vi "iWorx - Respiration Belt.vi"() -> ()   [LabVIEW 2012]
uses:
  <vilib>/measure/NI_MAPro.lvlib
  <vilib>/Analysis/NI_AALBase.lvlib
  <vilib>/Analysis/baseanly.llb/Mean (DBL).vi
  <vilib>/DAQmx/read.llb/DAQmx Read (Analog 1D Wfm NChan NSamp).vi
  <vilib>/DAQmx/configure/timing.llb/DAQmx Timing (Sample Clock).vi
  <vilib>/measure/macond.llb/IIR Filter for 1 Chan.vi
  <vilib>/DAQmx/create/channels.llb/DAQmx Create Channel (AI-Voltage-Basic).vi
panel:
  in  "Log Info Button":bool
  in  "Reset Scale":bool
  in  "Stop":bool
  out "Inst Breath Rate":dbl format="%5.1f BPM"
  in  "Set Up":bool
  in  "High Threshold":dbl=0.0005 format="%.5g"
  out "Avg Breath Rate":dbl format="%5.1f BPM"
  in  "Low Threshold":dbl=-0.0005 format="%.5f"
  out "error out":errorcluster
  in  "Auto-Threshold":bool
  in  "Channel":u16(ring) items=["Channel 1", "Channel 2"]
  in  "Pause Button":bool
  in  "Snapshot":bool
  out "Waveform Chart":waveform(dbl)(graph)
  in  "Clear Chart":bool
  in  "Open Log":bool
  in  "Rescale Y":bool
  out "Raw Signal":dbl(knob) scale=-0.1..0.1
  # "iWorx - Respiration Belt - Data Logger"
  # "Sensor Input"
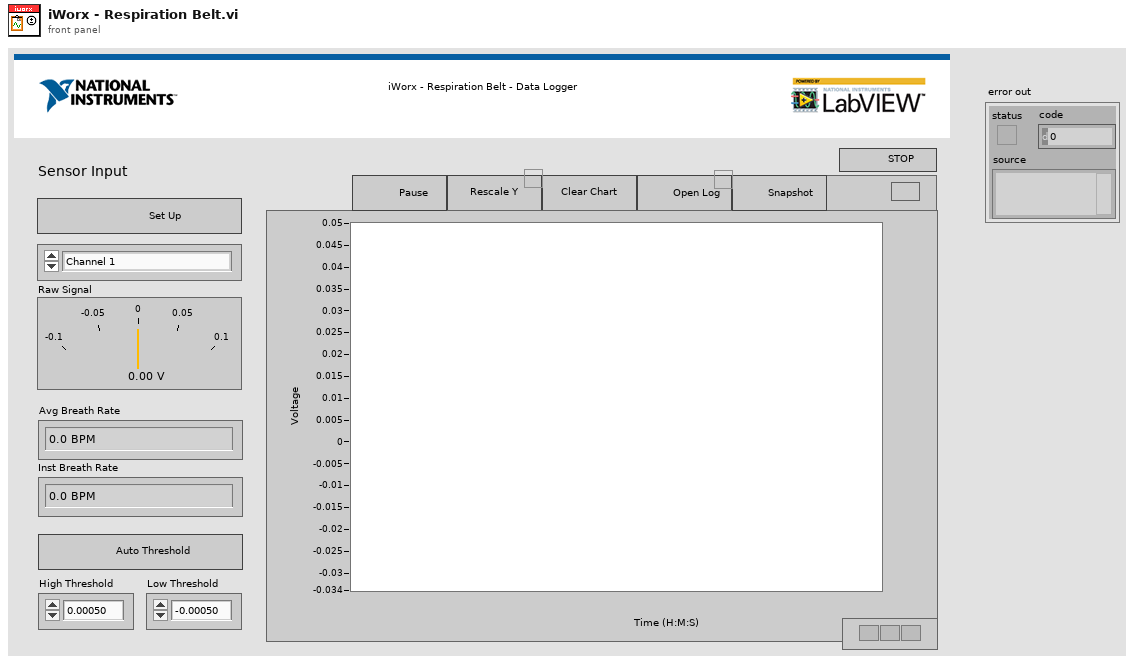
[diagram p1: front panel]
types:
  T1 = cluster{"Topology":enum16{"Off", "Butterworth", "Chebyshev", "Inverse Chebyshev", "Elliptic", "Bessel"}, "Type":enum16{"Lowpass", "Highpass", "Bandpass", "Bandstop"}, "Order":i32, "Lower Fc":dbl, "Upper Fc":dbl, "PB Ripple":dbl, "SB Attenuation":dbl}
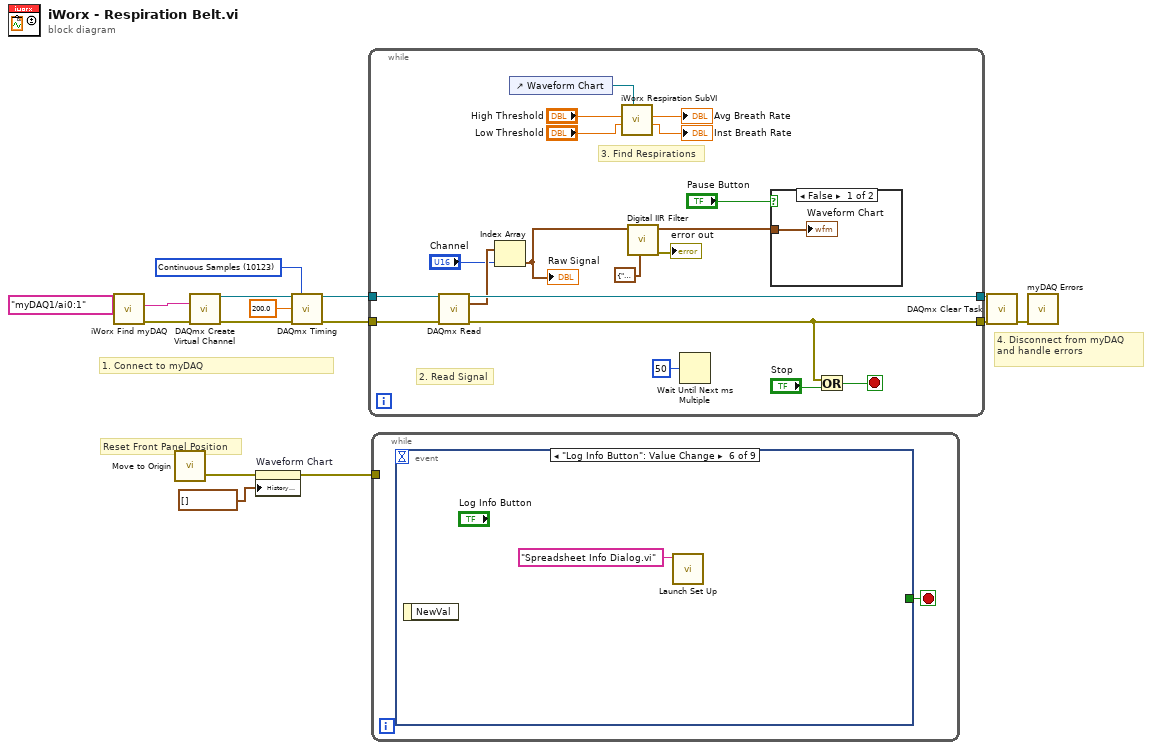
[diagram p0: block diagram]
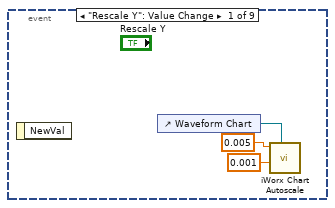
[diagram p2: hidden frame]
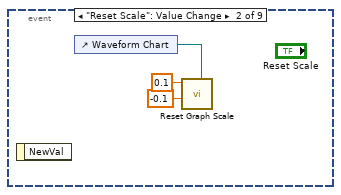
[diagram p3: hidden frame]
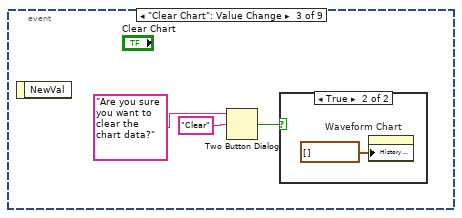
[diagram p4: hidden frame]
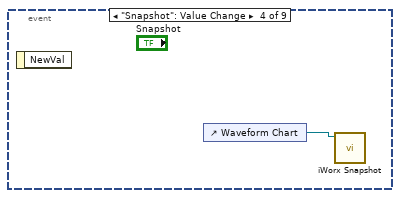
[diagram p6: hidden frame]
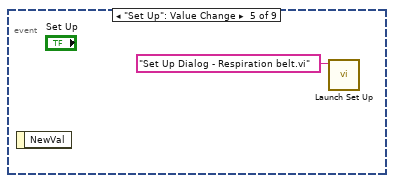
[diagram p7: hidden frame]
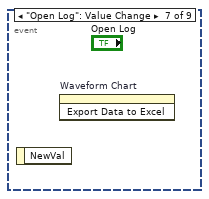
[diagram p8: hidden frame]
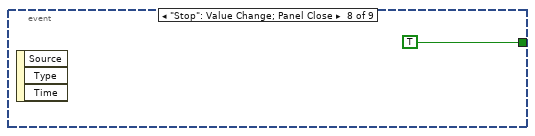
[diagram p9: hidden frame]
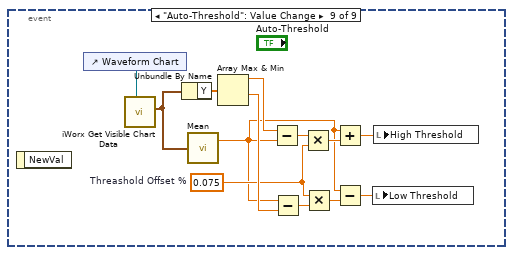
[diagram p10: hidden frame]
diagram:
  w7 = 10123 items=["Finite Samples"=10178, "Continuous Samples"=10123, "Hardware Timed Single Point"=12522] ("sample mode")
  # "Reset Front Panel Position"
  # "4. Disconnect from myDAQ and handle errors"
  # "1. Connect to myDAQ"
  n1 = call "iWorx Find myDAQ.vi"("Preferred myDAQ (myDAQ1)"=tag "myDAQ1/ai0:1" ("physical channels")) -> ("Error Out"=w3:errorcluster, "DAQmx Physical Channel"=w4:tag)  [unwired: 6 in, 3 out]
  n2 = call "Move to Origin.vi"() -> ("Error Out"=w2:errorcluster)  [unwired: 3 in]
  n3 = call-poly <vilib>:"DAQmx Create Virtual Channel.vi"("physical channels"=w4, "error in"=w3) -> ("task out"=w11:refnum<k21>, "error out"=w10:errorcluster)  [unwired: 12 in]
  n4 = property on="Waveform Chart" class="WFChart (strict)"(error in=w2, "History Data"=waveform(dbl)[] []) -> (error out=w13:errorcluster)  [unwired: 1 in, 1 out]
  n5 = call-poly <vilib>:"DAQmx Timing.vi"("task/channels in"=w11, "sample mode"=w7, "rate"=200.0, "error in"=w10) -> ("task out"=w8:refnum<k21>, "error out"=w9:errorcluster)  [unwired: 10 in]
  n6 = while {
    tunnel: w8 -> [w34]
    tunnel: [w33] -> w15
    tunnel: w9 -> [w32]
    tunnel: [w30] -> w14
    stop <- w31 stop-if-true
    # "3. Find Respirations"
    # "2. Read Signal"
    n7 = call-poly <vilib>:"DAQmx Read.vi"("task/channels in"=w34, "error in"=w32) -> ("task out"=w33:refnum<k21>, "data"=w28:waveform(dbl)[], "error out"=w30:errorcluster)  [unwired: 11 in]
    n8 = Index Array(array=w28, index="Channel") -> (element=w17:waveform(dbl))
    "Raw Signal" <- w17
    n9 = control-ref of="Waveform Chart"() -> (w22:refnum<vi>)
    n10 = call "iWorx Respiration SubVI.vi"("Waveform Chart"=w22, "low Threshold"="Low Threshold", "high Threshold"="High Threshold") -> ("Instantaneous Breath Rate"=→"Inst Breath Rate":dbl, "Avg Breaths per Minute"=→"Avg Breath Rate":dbl)  [unwired: 5 in, 2 out]
    n11 = call-poly <vilib>:"Digital IIR Filter.vi"("IIR filter specifications"=T1 {"Topology"=enum."Butterworth", "Type"=enum."Lowpass", "Order"=1, "Lower Fc"=1.0, "Upper Fc"=200.0, "PB Ripple"=1.0, "SB Attenuation"=60.0}, "signal in"=w17) -> ("error out"=→"error out":errorcluster, "signal out"=w23:waveform(dbl))  [unwired: 7 in, 1 out]
    n12 = Wait Until Next ms Multiple(millisecond multiple=u32 50) -> ()  [unwired: 1 out]
    n13 = case shown="False" "Pause Button" {
      tunnel: w23 -> [w35 _]
      frame False {
        "Waveform Chart" <- w35
      }
      frame True {
      }
    }
    n14 = Or(x=w30, y="Stop") -> (x .or. y?=w31:bool)
  }
  n15 = while {
    tunnel: w13 -> [_]
    stop <- w36 stop-if-true
    n16 = event shown="[5] \"Log Info Button\": Value Change" {
      selector: _ -> [_ _ _ _ _ _ _ _ _]
      dyn-events: _ -> [_ _ _ _ _ _ _ _ _]
      timeout: _ -> [_ _ _ _ _ _ _ _ _]
      tunnel: [_ _ _ _ _ _ _ TRUE _] -> w36
      event "Rescale Y": Value Change {
        n17 = event-data() -> ()  [unwired: 1 in, 1 out]
        n18 = control-ref of="Waveform Chart"() -> (w39:refnum<vi>)
        n19 = call "iWorx Chart Autoscale.vi"("Selection Chart"=w39, "Rounding Multiple (10)"=0.001 ("Rounding Multiple (1)"), "Min Range (1)"=0.005 ("Rounding Multiple (1)")) -> ()  [unwired: 6 in, 3 out]
      }
      event "Reset Scale": Value Change {
        n20 = event-data() -> ()  [unwired: 1 in, 1 out]
        n21 = control-ref of="Waveform Chart"() -> (w40:refnum<vi>)
        n22 = call "Reset Graph Scale.vi"("WaveformChart in"=w40, "Minimum (0)"=-0.1, "Maximum (100)"=0.1) -> ()  [unwired: 8 in, 1 out]
      }
      event "Clear Chart": Value Change {
        n23 = event-data() -> ()  [unwired: 1 in, 1 out]
        n24 = Two Button Dialog(message="Are you sure you want to clear the chart data?", 2:"Clear" ("T button name (\"OK\")")) -> (T button?=w44:bool)  [unwired: 1 in]
        n25 = case shown="True" w44 {
          frame False {
          }
          frame True {
            n26 = property on="Waveform Chart" class="WFChart (strict)"("History Data"=waveform(dbl)[] []) -> ()  [unwired: 2 in, 2 out]
          }
        }
      }
      event "Snapshot": Value Change {
        n27 = event-data() -> ()  [unwired: 1 in, 1 out]
        n28 = control-ref of="Waveform Chart"() -> (w47:refnum<vi>)
        n29 = call "iWorx Snapshot.vi"("WaveformChart in"=w47) -> ()  [unwired: 10 in, 1 out]
      }
      event "Set Up": Value Change {
        n30 = event-data() -> ()  [unwired: 1 in, 1 out]
        n31 = call "Launch Set Up.vi"("name or relative path"="Set Up Dialog - Respiration belt.vi") -> ()  [unwired: 9 in, 2 out]
      }
      event "Log Info Button": Value Change {
        n32 = event-data() -> ()  [unwired: 1 in, 1 out]
        n33 = call "Launch Set Up.vi"("name or relative path"="Spreadsheet Info Dialog.vi") -> ()  [unwired: 9 in, 2 out]
      }
      event "Open Log": Value Change {
        n34 = event-data() -> ()  [unwired: 1 in, 1 out]
        n35 = invoke on="Waveform Chart" class="WFChart (strict)" method="Export Data to Excel"() -> ()  [unwired: 3 in, 3 out]
      }
      event "Stop": Value Change; Panel Close {
        n36 = event-data() -> ()  [unwired: 1 in, 3 out]
      }
      event "Auto-Threshold": Value Change {
        w55 = 0.075  # Threashold Offset %
        n37 = event-data() -> ()  [unwired: 1 in, 1 out]
        n38 = control-ref of="Waveform Chart"() -> (w63:refnum<vi>)
        n39 = call "iWorx Get Visible Chart Data.vi"("Selection Chart"=w63) -> ("Waveform out"=w62:waveform(dbl))  [unwired: 8 in, 2 out]
        n40 = Unbundle By Name(w62) -> ("Y"=w61:dbl[])
        n41 = call-poly <vilib>:"Mean.vi"("X"=w62) -> ("mean"=w54:dbl)  [unwired: 1 out]
        n42 = Array Max & Min(array=w61) -> (max value=w60:dbl, min value=w57:dbl)  [unwired: 2 out]
        n43 = Subtract(x=w60, y=w54) -> (x-y=w59:dbl)
        n44 = Subtract(x=w54, y=w57) -> (x-y=w56:dbl)
        n45 = Multiply(x=w59, y=w55) -> (x*y=w58:dbl)
        n46 = Multiply(x=w55, y=w56) -> (x*y=w53:dbl)
        n47 = Add(x=w54, y=w58) -> (x+y=w52:dbl)
        n48 = Subtract(x=w54, y=w53) -> (x-y=w51:dbl)
        n49 = local write "Low Threshold"(w51) -> ()
        n50 = local write "High Threshold"(w52) -> ()
      }
    }
  }
  n51 = call <vilib>:"DAQmx Clear Task.vi"("task in"=w15, "error in"=w14) -> ("error out"=w1:errorcluster)  [unwired: 13 in]
  n52 = call "myDAQ Errors.vi"("error in (no error)"=w1) -> ()  [unwired: 10 in, 1 out]
